vi "_094.vi"() -> ()   [LabVIEW 2020]
panel:
  out "Array 2":i32[](array[numeric])
  out "Iteration outer loop":i32
  out "x+1 2":i32
  out "Array":i32[][](array[numeric])
  out "x+1":i32
  # "For Loop Logics :"
  # "Inner Loop :"
  # "Outer Loop :"
  # "The inner loop will run 7 times with the each count of the outer Loop ."
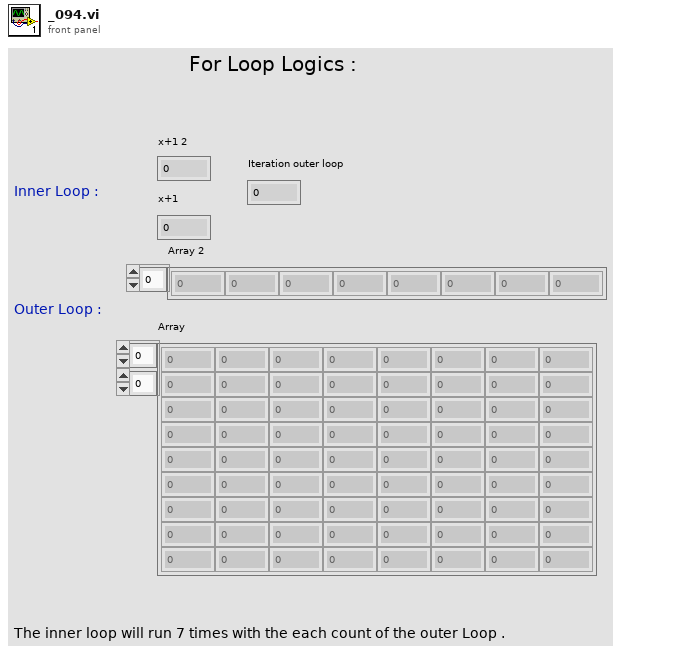
[diagram p1: front panel]
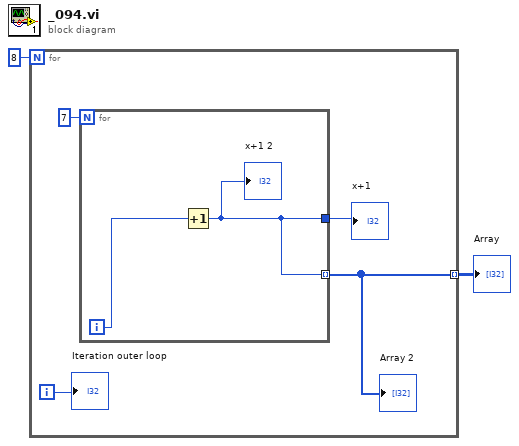
[diagram p0: block diagram]
diagram:
  n1 = for {
    N: 8 -> [_]
    tunnel: [w3] -> w1 mode=indexing
    i -> [w4]
    n2 = for {
      N: 7 -> [_]
      tunnel: [w7] -> w5
      tunnel: [w7] -> w3 mode=indexing
      i -> [w8]
      n3 = Increment(x=w8) -> (x+1=w7:i32)
      "x+1 2" <- w7
    }
    "x+1" <- w5
    "Array 2" <- w3
    "Iteration outer loop" <- w4
  }
  "Array" <- w1
